vi "Load Plugin Subpanel.vi"(8 "error in (no error)":errorcluster, 9 "Plugin Name":string, 10 "Path":path, 11 "CIF_UI in":refnum<class "CIF_UI.lvclass">) -> (0 "error out":errorcluster, 2 "VI Reference":refnum<vi>, 3 "CIF_UI out":refnum<class "CIF_UI.lvclass">)   [LabVIEW 2021, in "CIF_UI.lvclass"]
uses:
  CIF_UI.lvclass
  Typedef/Subpanel Data.ctl
  Typedef/Plugin Subpanel Events.ctl
  CIF_UI.lvclass/CIF_UI.ctl
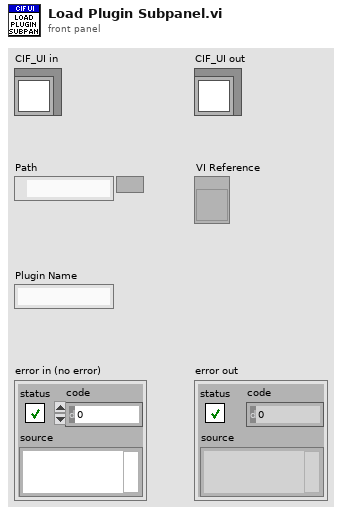
[diagram p1: front panel]
types:
  T1 = typedef "CIF_UI.lvclass/Subpanel Data.ctl" = cluster{"VI Reference":refnum<vi>, "Plugin Subpanel Events":T2}
  T2 = typedef "CIF_UI.lvclass/Plugin Subpanel Events.ctl" = cluster{"Plugin Shutdown":refnum<user-event>}
  T3 = typedef "CIF_UI.lvclass/Class Data for SubPanel.ctl" = cluster{"IP Address":string, "Server Certificate File (.crt)":path, "Connected":bool, "Core UI References":T4, "Subpanel Events":T5, "Manager gRPC Port":u16}
  T4 = typedef "CIF_UI.lvclass/Core UI References.ctl" = cluster{"Plugin Status":refnum<vi>, "Plugin Status Valid":bool, "Connection":refnum<vi>, "Connection Valid":bool, "Exit":refnum<vi>, "Exit Valid":bool, "Run Listen":refnum<vi>, "Run Listen Valid":bool, "Clear Local Error":refnum<vi>, "Clear Local Error Valid":bool, "Local Error":refnum<vi>, "Local Error Valid":bool}
  T5 = typedef "CIF_UI.lvclass/SubPanel Events.ctl" = cluster{"Clear Local Error":refnum<user-event>, "Shutdown":refnum<user-event>, "Plugin Connection":refnum<user-event>}
  T6 = typedef "CIF_UI.lvclass/Plugin Subpanel Map.ctl" = map{i32, T1}
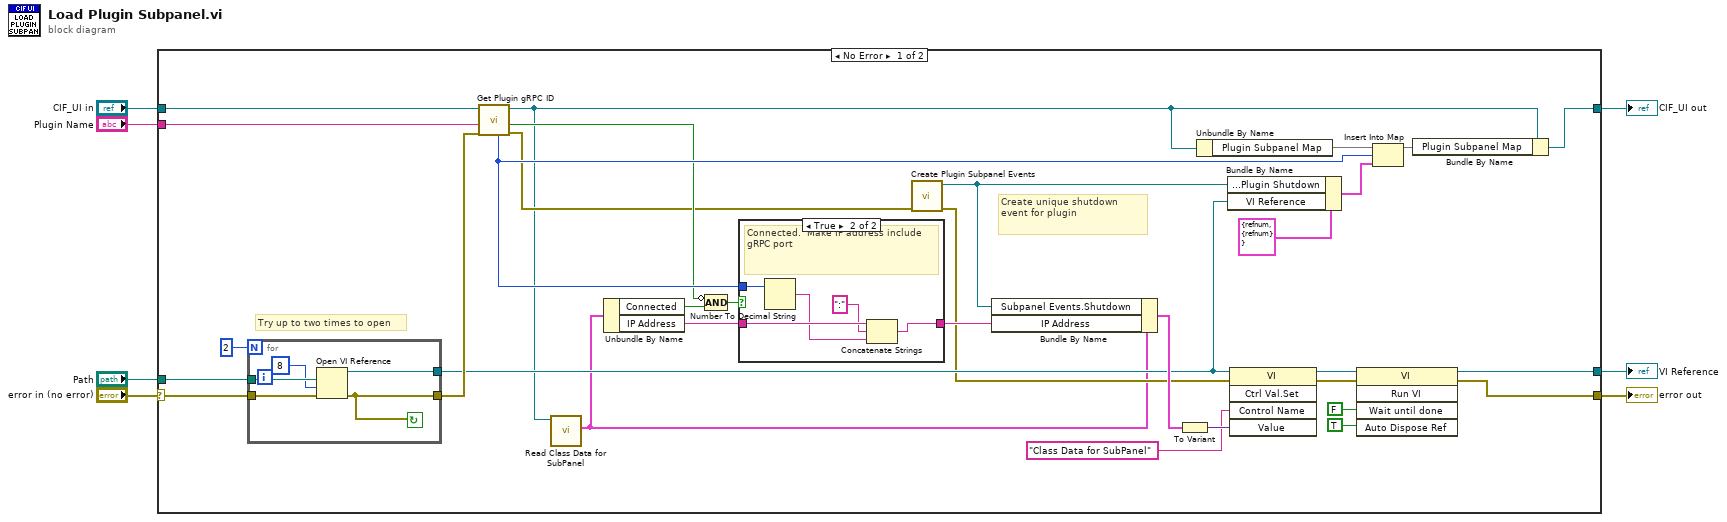
[diagram p0: block diagram]
diagram:
  n1 = case shown="No Error" "error in (no error)" {
    selector: "error in (no error)" -> [w31 w52]
    tunnel: [w30 w52] -> w6
    tunnel: [w9 w51] -> w5
    tunnel: "CIF_UI in" -> [w26 w51]
    tunnel: [w28 _] -> w4
    tunnel: "Path" -> [w27 _]
    tunnel: "Plugin Name" -> [w25 _]
    frame No Error {
      # "Create unique shutdown event for plugin"
      # "Try up to two times to open"
      n2 = for {
        N: 2 -> [_]
        tunnel: w27 -> [w50]
        tunnel: [w49] -> w13
        tunnel: [w46] -> w24
        tunnel: w31 -> [w47]
        stop <- w46 continue-if-true
        n3 = Open VI Reference(vi path=w50, options=8, error in (no error)=w47) -> (vi reference=w49:refnum<vi>, error out=w46:errorcluster)  [unwired: 3 in]
      }
      n4 = call "Get Plugin gRPC ID.vi"("error in (no error)"=w24, "Plugin Name"=w25, "CIF_UI in"=w26) -> ("error out"=w16:errorcluster, "Not Found"=w18:bool, "CIF_UI out"=w10:refnum<class "CIF_UI.lvclass">, "gRPC Port"=w20:i32)  [unwired: 4 in, 1 out]
      n5 = call "Read Class Data for SubPanel.vi"("CIF_UI in"=w10) -> ("Class Data for SubPanel"=w8:T3)  [unwired: 8 in, 2 out]
      n6 = Unbundle By Name(w8) -> ("Connected"=w19:bool, "IP Address"=w23:string)
      n7 = Compound Arithmetic op=AND(invert w18, w19) -> (w17:bool)
      n8 = case shown="True" w17 {
        tunnel: w23 -> [w40 w44]
        tunnel: [w40 w41] -> w21
        tunnel: w20 -> [_ w45]
        frame False {
          # "Not connected"
        }
        frame True {
          # "Connected.  Make IP address include gRPC port"
          n9 = Number To Decimal String(number=w45) -> (decimal integer string=w43:string)  [unwired: 1 in]
          n10 = Concatenate Strings(w44, ":" ("string"), w43) -> (w41:string)
        }
      }
      n11 = call "Create Plugin Subpanel Events.vi"("error in (no error)"=w16) -> ("error out"=w12:errorcluster, "Plugin Shutdown Event"=w11:refnum<user-event>)  [unwired: 9 in]
      n12 = Bundle By Name(cluster=w8, "Subpanel Events.Shutdown"=w11, "IP Address"=w21) -> (w22:T3)
      n13 = To Variant(anything=w22) -> (Variant=w35:variant)
      n14 = Unbundle By Name(w10) -> ("Plugin Subpanel Map"=w33:T6)
      n15 = Bundle By Name(cluster=T1 {"VI Reference"=refnum, "Plugin Subpanel Events"={"Plugin Shutdown"=refnum}} ("SubPanel Data"), "Plugin Subpanel Events.Plugin Shutdown"=w11, "VI Reference"=w13) -> (w32:T1)
      n16 = invoke class="VI" method="Ctrl Val.Set"(reference=w13, error in=w12, "Control Name"="Class Data for SubPanel", "Value"=w35) -> (reference out=w14:refnum<vi>, error out=w15:errorcluster)  [unwired: 1 in, 3 out]
      n17 = invoke class="VI" method="Run VI"(reference=w14, error in=w15, "Wait until done"=FALSE ("Wait Until Done"), "Auto Dispose Ref"=TRUE ("Auto Dispose Reference")) -> (reference out=w28:refnum<vi>, error out=w30:errorcluster)  [unwired: 1 in, 3 out]
      n18 = Insert Into Map(map in=w33, key=w20, value=w32) -> (map out=w29:T6)  [unwired: 2 out]
      n19 = Bundle By Name(cluster=w10, "Plugin Subpanel Map"=w29) -> (w9:refnum<class "CIF_UI.lvclass">)
    }
    frame Error {
    }
  }
  "error out" <- w6
  "CIF_UI out" <- w5
  "VI Reference" <- w4
